vi "Get Digest.vi"(11 "Hash Function in":refnum<class "NI_SHA-512.lvclass">) -> (2 "digest":u8[](array[numeric]) format="%02x", 3 "Hash Function out":refnum<class "NI_SHA-512.lvclass">)   [LabVIEW 2020, in "NI_SHA-512.lvclass"]
doc: "Compute the message digest given previously supplied input blocks."
uses:
  <vilib>/security/Message Digest/SHA-2/SHA-512/NI_SHA-512.lvclass
  <vilib>/security/Message Digest/SHA-2/SHA-512/NI_SHA-512.lvclass/NI_SHA-512.ctl
  <vilib>/Bit Manipulation/wrappers/Words To Network-Order Bytes/Words To Network-Order Bytes U64.vi
  <vilib>/Bit Manipulation/NI_Bit Manipulation.lvlib
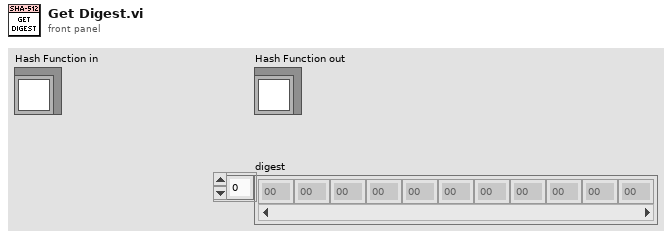
[diagram p1: front panel]
types:
  T1 = typedef "NI_SHA-512.lvclass/Mode.ctl" = enum16{"SHA-512", "SHA-384", "SHA-512/256", "SHA-512/224"}
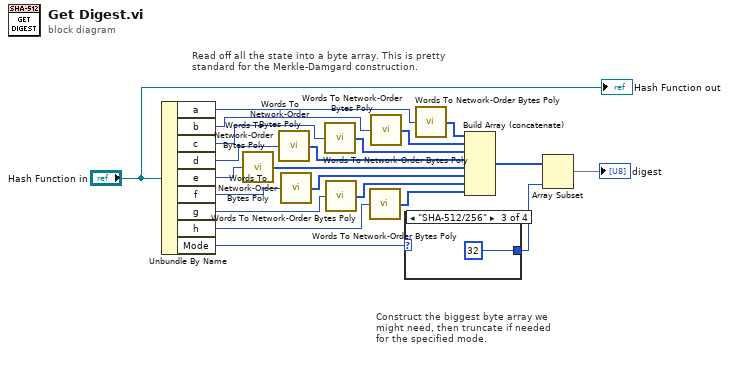
[diagram p0: block diagram]
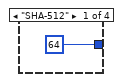
[diagram p2: hidden frame]
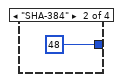
[diagram p3: hidden frame]
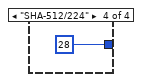
[diagram p4: hidden frame]
diagram:
  # "Construct the biggest byte array we might need, then truncate if needed for the specified mode."
  # "Read off all the state into a byte array. This is pretty standard for the Merkle-Damgard construction."
  n1 = Unbundle By Name("Hash Function in") -> ("a"=w19:u64, "b"=w17:u64, "c"=w16:u64, "d"=w15:u64, "e"=w14:u64, "f"=w13:u64, "g"=w12:u64, "h"=w11:u64, "Mode"=w1:T1)
  n2 = call-poly <vilib>:"Words To Network-Order Bytes Poly.vi"("word"=w14) -> ("bytes"=w7:u8[])
  n3 = call-poly <vilib>:"Words To Network-Order Bytes Poly.vi"("word"=w15) -> ("bytes"=w6:u8[])
  n4 = call-poly <vilib>:"Words To Network-Order Bytes Poly.vi"("word"=w13) -> ("bytes"=w8:u8[])
  n5 = call-poly <vilib>:"Words To Network-Order Bytes Poly.vi"("word"=w16) -> ("bytes"=w5:u8[])
  n6 = call-poly <vilib>:"Words To Network-Order Bytes Poly.vi"("word"=w12) -> ("bytes"=w9:u8[])
  n7 = call-poly <vilib>:"Words To Network-Order Bytes Poly.vi"("word"=w11) -> ("bytes"=w10:u8[])
  n8 = call-poly <vilib>:"Words To Network-Order Bytes Poly.vi"("word"=w17) -> ("bytes"=w4:u8[])
  n9 = case shown="\"SHA-512/256\"" w1 {
    tunnel: [64 ("length") 48 ("length") 32 ("length") 28 ("length")] -> w20
    frame "SHA-512" {
    }
    frame "SHA-384" {
    }
    frame "SHA-512/256" {
    }
    frame "SHA-512/224" {
    }
  }
  n10 = call-poly <vilib>:"Words To Network-Order Bytes Poly.vi"("word"=w19) -> ("bytes"=w18:u8[])
  n11 = Build Array (concatenate)(w18, w4, w5, w6, w7, w8, w9, w10) -> (w2:u8[])
  n12 = Array Subset(array=w2, length=w20) -> (→"digest":u8[])  [unwired: 1 in]
  "Hash Function out" <- "Hash Function in"
